vi "Read Index.vi"(8 "error in (no error)":errorcluster, 11 "CCD in":refnum<class "CCD.lvclass">) -> (0 "error out":errorcluster, 2 "Index":i32, 3 "CCD out":refnum<class "CCD.lvclass">)   [LabVIEW 2023, in "CCD.lvclass"]
uses:
  CCD.lvclass
  GenericDevice/GenericDevice.lvclass
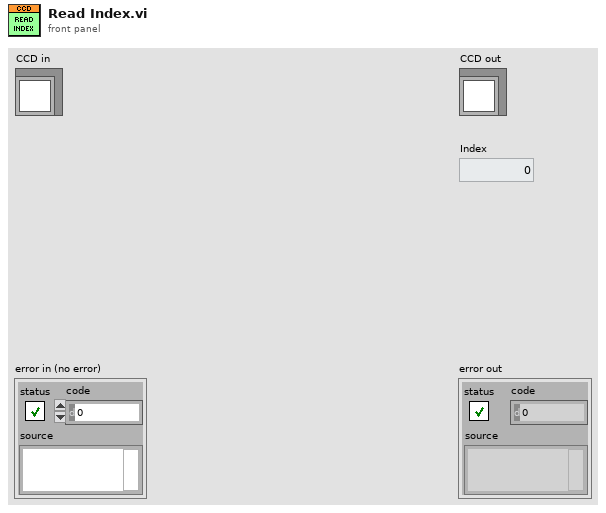
[diagram p1: front panel]
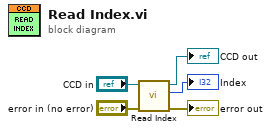
[diagram p0: block diagram]
diagram:
  n1 = call-parent "Read Index.vi"("error in (no error)"="error in (no error)", "GenericDevice in"="CCD in") -> ("error out"=→"error out":errorcluster, "Index"=→"Index":i32, "GenericDevice out"=→"CCD out":refnum<class "CCD.lvclass">)  [unwired: 7 in]
